vi "Tach Hysteresis Analog (No State).vi"(0 "input signal":sgl[](array[numeric]), 1 "reset? (T)":bool=TRUE, 5 "threshold (auto)":sgl=inf format="%.2f", 7 "slope (Rising)":u16(ring) items=["Rising", "Falling"], 9 "hysteresis(0)":sgl format="%.2f", 11 "error in (no error)":errorcluster, 12 "last value in":sgl) -> (4 "output signal":sgl[](array[numeric]), 14 "last value out":sgl, 15 "error out":errorcluster)   [LabVIEW 2017, in "VibrationAnalysisFunctions.lvlib"]
doc: "This VI works like a hysteresis comparater. It can transform the input tachometer signal into a standard square waveform, ignoring small pulsed caused by harmonics or noise. By setting the hystersis value properly, it can make the speed tracking more accurately."
uses:
  <vilib>/addons/InsightCM/Utilities/Analysis/Vibration/VibrationAnalysisFunctions.lvlib
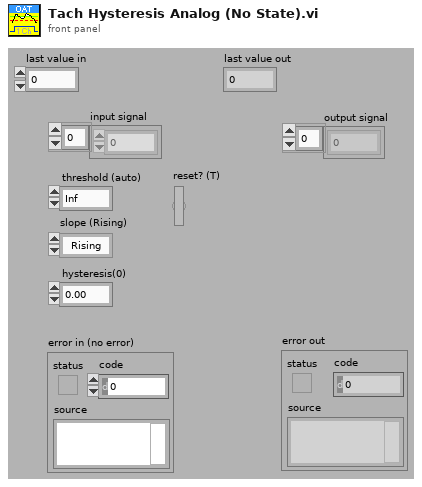
[diagram p1: front panel]
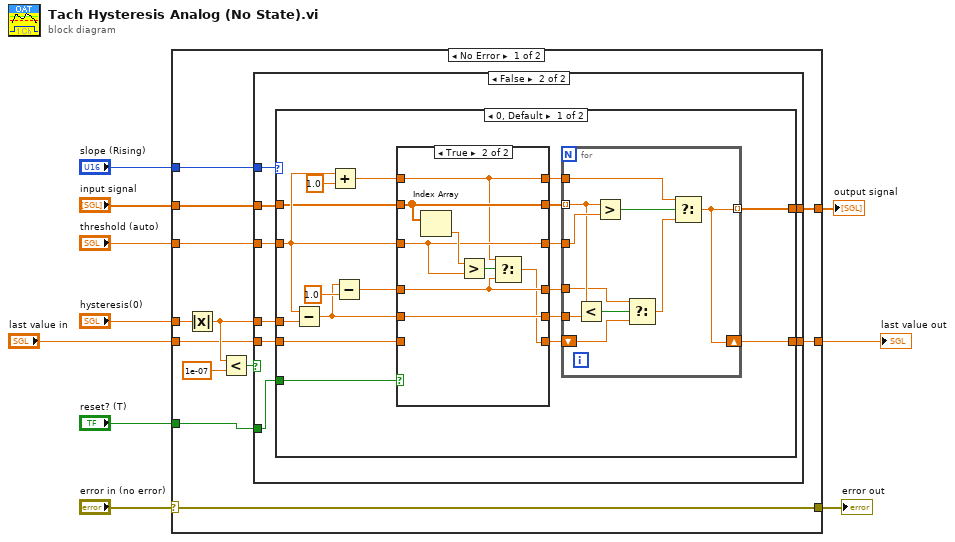
[diagram p0: block diagram]
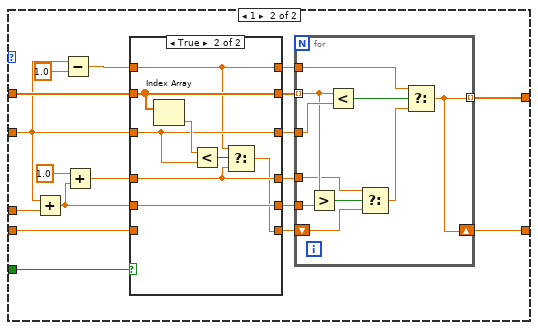
[diagram p4: hidden frame]
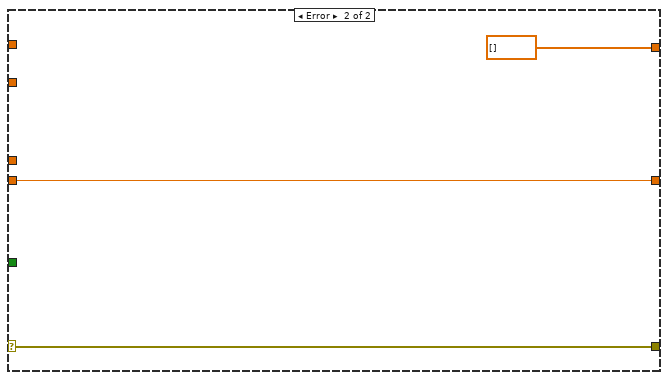
[diagram p6: hidden frame]
diagram:
  n1 = case shown="No Error" "error in (no error)" {
    selector: "error in (no error)" -> [w18 w119]
    tunnel: "reset? (T)" -> [w13 _]
    tunnel: "hysteresis(0)" -> [w14 _]
    tunnel: "threshold (auto)" -> [w21 _]
    tunnel: "slope (Rising)" -> [w20 _]
    tunnel: [w19 sgl[] [] ("signal")] -> w3
    tunnel: [w18 w119] -> w5
    tunnel: "input signal" -> [w17 _]
    tunnel: "last value in" -> [w12 w117]
    tunnel: [w11 w117] -> w1
    frame No Error {
      n2 = Absolute Value(x=w14) -> (abs(x)=w15:sgl)
      n3 = Less?(x=w15, y=1e-07) -> (x < y?=w22:bool)
      n4 = case shown="False" w22 {
        tunnel: w17 -> [w24 w29]
        tunnel: [w24 w28] -> w19
        tunnel: w15 -> [_ w27]
        tunnel: w20 -> [_ w32]
        tunnel: w21 -> [_ w31]
        tunnel: w13 -> [_ w30]
        tunnel: w12 -> [w23 w26]
        tunnel: [w23 w25] -> w11
        frame True {
        }
        frame False {
          n5 = case shown="0, Default" w32 {
            tunnel: w29 -> [w43 w92]
            tunnel: w31 -> [w45 w88]
            tunnel: w27 -> [w49 w89]
            tunnel: w30 -> [w42 w83]
            tunnel: [w41 w84] -> w28
            tunnel: w26 -> [w40 w82]
            tunnel: [w39 w81] -> w25
            frame 0, Default {
              n6 = Subtract(x=w45, y=w49) -> (x-y=w47:sgl)
              n7 = Add(x=w45, y=sgl 1.0) -> (x+y=w44:sgl)
              n8 = Subtract(x=w47, y=sgl 1.0) -> (x-y=w48:sgl)
              n9 = case shown="True" w42 {
                tunnel: w47 -> [w55 w64]
                tunnel: [w55 w64] -> w38
                tunnel: w48 -> [w54 w58]
                tunnel: [w54 w58] -> w37
                tunnel: w45 -> [w53 w61]
                tunnel: [w53 w61] -> w36
                tunnel: w43 -> [w52 w63]
                tunnel: [w52 w63] -> w35
                tunnel: w44 -> [w51 w59]
                tunnel: [w51 w59] -> w34
                tunnel: w40 -> [w56 _]
                tunnel: [w56 w57] -> w33
                frame False {
                }
                frame True {
                  n10 = Index Array(array=w63) -> (element=w62:sgl)  [unwired: 1 in]
                  n11 = Greater?(x=w62, y=w61) -> (0:w60:bool)
                  n12 = Select(t=w59, s=w60, f=w58) -> (s? t:f=w57:sgl)
                }
              }
              n13 = for {
                tunnel: w35 -> [w72] mode=indexing
                tunnel: w36 -> [w74]
                shift-right: [w65] -> w39
                shift-left: w33 -> [w66]
                tunnel: w38 -> [w70]
                tunnel: w34 -> [w69]
                tunnel: w37 -> [w67]
                tunnel: [w65] -> w41 mode=indexing
                n14 = Less?(x=w72, y=w70) -> (x < y?=w71:bool)
                n15 = Greater?(x=w72, y=w74) -> (0:w73:bool)
                n16 = Select(t=w67, s=w71, f=w66) -> (s? t:f=w68:sgl)
                n17 = Select(t=w69, s=w73, f=w68) -> (s? t:f=w65:sgl)
              }
            }
            frame 1 {
              n18 = Add(x=w88, y=w89) -> (x+y=w85:sgl)
              n19 = Subtract(x=w88, y=sgl 1.0) -> (x-y=w91:sgl)
              n20 = Add(x=sgl 1.0, y=w85) -> (x+y=w86:sgl)
              n21 = case shown="True" w83 {
                tunnel: w85 -> [w97 w106]
                tunnel: [w97 w106] -> w80
                tunnel: w86 -> [w96 w100]
                tunnel: [w96 w100] -> w79
                tunnel: w88 -> [w95 w103]
                tunnel: [w95 w103] -> w78
                tunnel: w92 -> [w94 w105]
                tunnel: [w94 w105] -> w77
                tunnel: w91 -> [w93 w101]
                tunnel: [w93 w101] -> w76
                tunnel: w82 -> [w98 _]
                tunnel: [w98 w99] -> w75
                frame False {
                }
                frame True {
                  n22 = Index Array(array=w105) -> (element=w104:sgl)  [unwired: 1 in]
                  n23 = Less?(x=w104, y=w103) -> (x < y?=w102:bool)
                  n24 = Select(t=w101, s=w102, f=w100) -> (s? t:f=w99:sgl)
                }
              }
              n25 = for {
                tunnel: w77 -> [w114] mode=indexing
                tunnel: w78 -> [w116]
                shift-right: [w107] -> w81
                shift-left: w75 -> [w108]
                tunnel: w80 -> [w112]
                tunnel: w76 -> [w111]
                tunnel: w79 -> [w109]
                tunnel: [w107] -> w84 mode=indexing
                n26 = Greater?(x=w114, y=w112) -> (0:w113:bool)
                n27 = Less?(x=w114, y=w116) -> (x < y?=w115:bool)
                n28 = Select(t=w109, s=w113, f=w108) -> (s? t:f=w110:sgl)
                n29 = Select(t=w111, s=w115, f=w110) -> (s? t:f=w107:sgl)
              }
            }
          }
        }
      }
    }
    frame Error {
    }
  }
  "error out" <- w5
  "output signal" <- w3
  "last value out" <- w1
